vi "PingTestCore.vi"(8 "error in (no error)":errorcluster, 10 "Timeout ms":i32=1000, 11 "IpAdress in":string) -> (0 "error out":errorcluster, 3 "Failed?":bool)   [LabVIEW 2014]
uses:
  <vilib>/regexp/Match Regular Expression.xnode
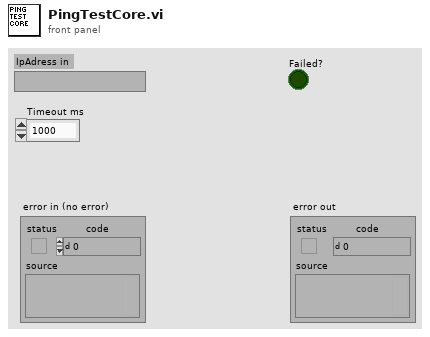
[diagram p1: front panel]
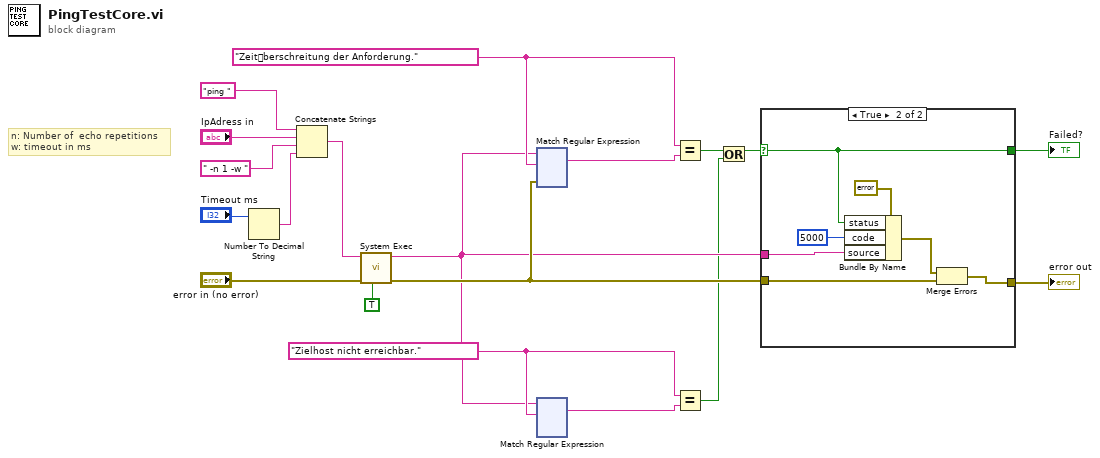
[diagram p0: block diagram]
diagram:
  w9 = "Zielhost nicht erreichbar." ("regular expression")
  w17 = "Zeitberschreitung der Anforderung." ("regular expression")
  # "n: Number of  echo repetitions\nw: timeout in ms"
  n1 = Number To Decimal String(number="Timeout ms") -> (decimal integer string=w1:string)  [unwired: 1 in]
  n2 = Concatenate Strings("ping " ("string"), "IpAdress in", " -n 1 -w " ("string"), w1) -> (w13:string)
  n3 = call <vilib>:"System Exec.vi"("run minimized? (F)"=TRUE, "error in (no error)"="error in (no error)", "command line"=w13) -> ("error out"=w15:errorcluster, "standard output"=w7:string)  [unwired: 5 in, 2 out]
  n4 = xnode "Match Regular Expression"("input string"=w7, "regular expression"=w17, "error in"=w15) -> ("whole match"=w18:string)  [unwired: 3 in, 4 out]
  n5 = xnode "Match Regular Expression"("input string"=w7, "regular expression"=w9) -> ("whole match"=w8:string)  [unwired: 4 in, 4 out]
  n6 = Equal?(x=w17, y=w18) -> (x = y?=w14:bool)
  n7 = Equal?(x=w9, y=w8) -> (x = y?=w5:bool)
  n8 = Or(x=w14, y=w5) -> (x .or. y?=w6:bool)
  n9 = case shown="True" w6 {
    selector: w6 -> [w20 w22]
    tunnel: [w21 w28] -> w16
    tunnel: w15 -> [w21 w27]
    tunnel: w7 -> [_ w24]
    tunnel: [w20 w22] -> w4
    frame False {
    }
    frame True {
      n10 = Bundle By Name(cluster=errorcluster {"status"=FALSE, "code"=0, "source"=""} ("error out"), "status"=w22, "code"=5000, "source"=w24) -> (w25:errorcluster)
      n11 = Merge Errors(w25, w27) -> (w28:errorcluster)
    }
  }
  "error out" <- w16
  "Failed?" <- w4
